vi "Menu_Cluster Wire.vi"(11 "Affected Items":T1) -> (3 "Menu Items To Add":T2(array[cluster]))   [LabVIEW 2023]
uses:
  top/BundleMagic.ctl
  controls/action enum.ctl
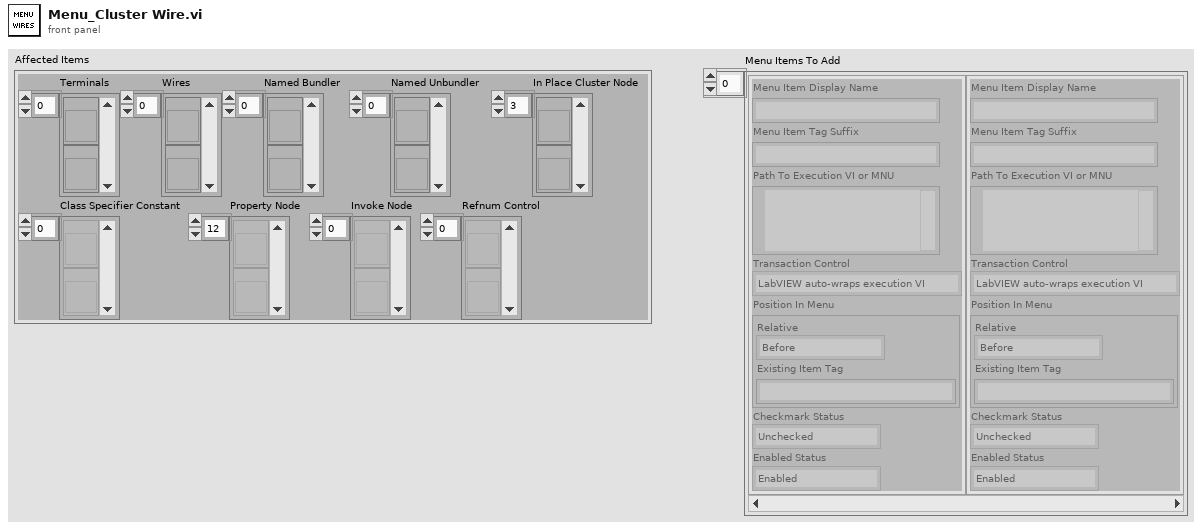
[diagram p1: front panel]
types:
  T1 = typedef "BundleMagic.ctl" = cluster{"Terminals":refnum<vi>[], "Wires":refnum<vi>[], "Named Bundler":refnum<vi>[], "Named Unbundler":refnum<vi>[], "In Place Cluster Node":refnum<vi>[], "Class Specifier Constant":refnum<vi>[], "Property Node":refnum<vi>[], "Invoke Node":refnum<vi>[], "Refnum Control":refnum<vi>[]}
  T2 = cluster{"Menu Item Display Name":string, "Menu Item Tag Suffix":string, "Path To Execution VI or MNU":path, "Transaction Control":enum8{"LabVIEW auto-wraps execution VI", "Execution VI will define if needed"}, "Position In Menu":cluster{"Relative":enum8{"Before", "Instead of", "After", "Into Submenu"}, "Existing Item Tag":string}, "Checkmark Status":enum8{"Unchecked", "Checked"}, "Enabled Status":enum8{"Enabled", "Disabled"}}[]
  T3 = typedef "action enum.ctl" = enum16{"[NONE]", "APP_SEPARATOR", "Wire Bundle", "Wire Unbundle", "Terminal Unbundle", "Terminal Bundle", "Bundler Move Up", "Bundler Move Down", "Bundler Insert", "Bundler Remove", "Bundler Remove Unwired", "Bundler Rearrange", "In Place Insert", "In Place Remove", "In Place Remove Unwired", "In Place Rearrange", "Wire Properties", "Wire Method", "Terminal Properties", "Terminal Method", "Property Move Up", "Property Move Down", "Properties Insert", "Properties Remove", "Properties Remove Unwired", "Properties Rearrange", "Method Change", "Class For Constant", "Class For Control", "Class For Node", "Class Name to Clipboard"}
  T4 = cluster{"Relative":enum8{"Before", "Instead of", "After", "Into Submenu"}, "Existing Item Tag":string}
  T5 = cluster{"Relative":enum8{"Before", "Instead of", "After", "Into Submenu"}, "Existing Item Tag":string}[]
  T6 = cluster{"Menu Item Display Name":string, "Menu Item Tag Suffix":string, "Path To Execution VI or MNU":path, "Transaction Control":enum8{"LabVIEW auto-wraps execution VI", "Execution VI will define if needed"}, "Position In Menu":cluster{"Relative":enum8{"Before", "Instead of", "After", "Into Submenu"}, "Existing Item Tag":string}, "Checkmark Status":enum8{"Unchecked", "Checked"}, "Enabled Status":enum8{"Enabled", "Disabled"}}
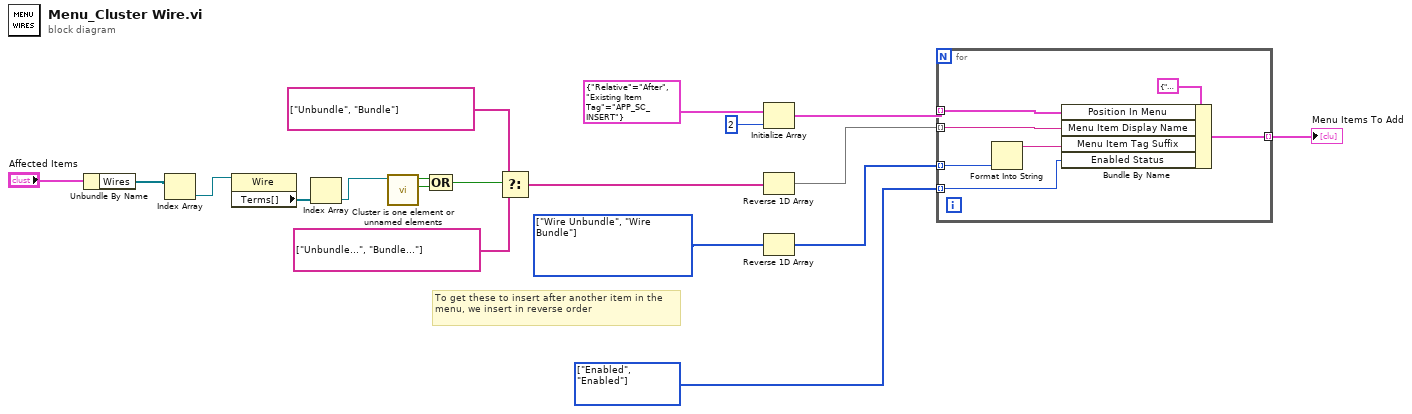
[diagram p0: block diagram]
diagram:
  w1 = T3[] [enum."Wire Unbundle", enum."Wire Bundle"] items=["[NONE]", "APP_SEPARATOR", "Wire Bundle", "Wire Unbundle", "Terminal Unbundle", "Terminal Bundle", "Bundler Move Up", "Bundler Move Down", "Bundler Insert", "Bundler Remove", "Bundler Remove Unwired", "Bundler Rearrange", "In Place Insert", "In Place Remove", "In Place Remove Unwired", "In Place Rearrange", "Wire Properties", "Wire Method", "Terminal Properties", "Terminal Method", "Property Move Up", "Property Move Down", "Properties Insert", "Properties Remove", "Properties Remove Unwired", "Properties Rearrange", "Method Change", "Class For Constant", "Class For Control", "Class For Node", "Class Name to Clipboard"] ("Array")
  w14 = enum8{"Enabled", "Disabled"}[] [enum."Enabled", enum."Enabled"] items=["Enabled", "Disabled"] ("Enabled Status")
  # "To get these to insert after another item in the menu, we insert in reverse order"
  n1 = Unbundle By Name("Affected Items") -> ("Wires"=w8:refnum<vi>[])
  n2 = Index Array(array=w8) -> (element=w7:refnum<vi>)  [unwired: 1 in]
  n3 = property class="Wire"(reference=w7) -> ("Terms[]"=w6:refnum<vi>[])  [unwired: 1 in, 2 out]
  n4 = Index Array(array=w6) -> (element=w5:refnum<vi>)  [unwired: 1 in]
  n5 = call "Cluster is one element or unnamed elements.vi"("Cluster Terminal"=w5) -> ("All Unnamed?"=w3:bool, "One Element?"=w4:bool)  [unwired: 8 in, 1 out]
  n6 = Compound Arithmetic op=OR(w4, w3) -> (w2:bool)
  n7 = Select(t=string[] ["Unbundle", "Bundle"], s=w2, f=string[] ["Unbundle...", "Bundle..."]) -> (s? t:f=w10:string[])
  n8 = Initialize Array(T4 {"Relative"=enum."After", "Existing Item Tag"="APP_SC_INSERT"} ("Position In Menu"), 2) -> (w13:T5)
  n9 = Reverse 1D Array(array=w10) -> (reversed array=w16:string[])
  n10 = Reverse 1D Array(array=w1) -> (reversed array=w15:T3[])
  n11 = for {
    tunnel: [w26] -> w17 mode=indexing
    tunnel: w16 -> [w25] mode=indexing
    tunnel: w15 -> [w20] mode=indexing
    tunnel: w13 -> [w23] mode=indexing
    tunnel: w14 -> [w22] mode=indexing
    n12 = Format Into String(w20) -> (resulting string=w21:string)  [unwired: 3 in, 1 out]
    n13 = Bundle By Name(cluster=T6 {"Menu Item Display Name"="", "Menu Item Tag Suffix"="", "Path To Execution VI or MNU"=path "", "Transaction Control"=enum."LabVIEW auto-wraps execution VI", "Position In Menu"={"Relative"=enum."Before", "Existing Item Tag"=""}, "Checkmark Status"=enum."Unchecked", "Enabled Status"=enum."Enabled"} ("Cluster"), "Position In Menu"=w23, "Menu Item Display Name"=w25, "Menu Item Tag Suffix"=w21, "Enabled Status"=w22) -> (w26:T6)
  }
  "Menu Items To Add" <- w17
